vi "Calculate B.vi"(10 "Frequency":dbl) -> (2 "B":dbl)   [LabVIEW 2014]
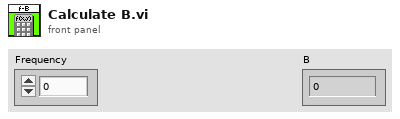
[diagram p1: front panel]
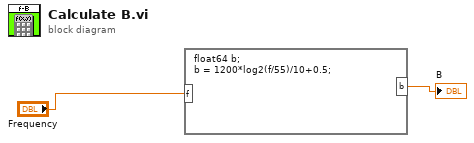
[diagram p0: block diagram]
diagram:
  n1 = formula code="float64 b;\nb = 1200*log2(f/55)/10+0.5;"("f"="Frequency") -> ("b"=→"B":dbl)
